vi "conversion_loop.vi"(0 "CAN frame array":T1[](array[typedef]) {"payload" format="%x"; "timestamp" format="%<%.7X\n%x>T"; "type" items=["CAN Data"=0, "CAN Remote"=1, "CAN Bus Error"=2, "CAN 2.0 Data"=8, "CAN FD Data"=16, "CAN FD+BRS Data"=24, "J1939 Data"=192, "Delay"=224, "Log Trigger"=225, "Start Trigger"=226]; "identifier" format="%x"}, 2 "CAN1 conversion session":T3, 3 "CAN2 conversion session":T3) -> (5 "CAN1 signal data":dbl[](array[numeric]), 6 "CAN2 signal data":dbl[](array[numeric]), 7 "CAN1 error out":errorcluster, 8 "CAN2 error out":errorcluster)   [LabVIEW 2017]
uses:
  <vilib>/xnet/xnet.llb/XNET Frame CAN.ctl
  <vilib>/xnet/xnet.llb/XNET Frame Type CAN.ctl
  <vilib>/xnet/xnet.llb/XNET Convert (Frame CAN to Signal).vi
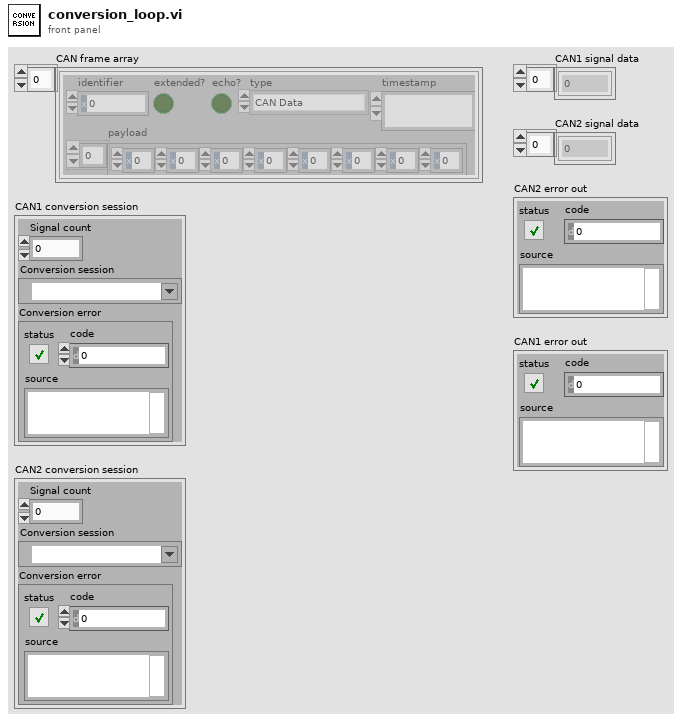
[diagram p1: front panel]
types:
  T1 = typedef "XNET Frame CAN.ctl" = cluster{"timestamp":timestamp, "payload":u8[], "identifier":u32, "type":T2, "extended?":bool, "echo?":bool}
  T2 = typedef "XNET Frame Type CAN.ctl" = u8
  T3 = cluster{"Signal count":i32, "Conversion session":refnum<k21>, "Conversion error":errorcluster}
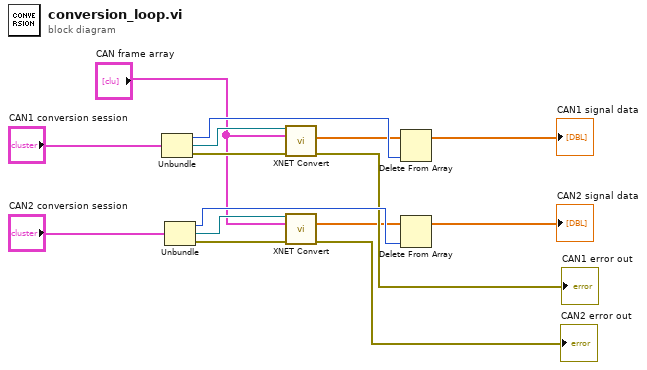
[diagram p0: block diagram]
diagram:
  n1 = Unbundle("CAN1 conversion session") -> ("Signal count"=w15:i32, "Conversion session"=w13:refnum<k21>, "Conversion error"=w10:errorcluster)
  n2 = Unbundle("CAN2 conversion session") -> ("Signal count"=w14:i32, "Conversion session"=w12:refnum<k21>, "Conversion error"=w11:errorcluster)
  n3 = call-poly <vilib>:"XNET Convert.vi"("session in"=w13, "frame data"="CAN frame array", "error in (no error)"=w10) -> ("signal data"=w1:dbl[], "error out"=→"CAN1 error out":errorcluster)  [unwired: 10 in, 1 out]
  n4 = call-poly <vilib>:"XNET Convert.vi"("session in"=w12, "frame data"="CAN frame array", "error in (no error)"=w11) -> ("signal data"=w2:dbl[], "error out"=→"CAN2 error out":errorcluster)  [unwired: 10 in, 1 out]
  n5 = Delete From Array(array=w1, index=w15) -> (array with subset deleted=→"CAN1 signal data":dbl[])  [unwired: 1 in, 1 out]
  n6 = Delete From Array(array=w2, index=w14) -> (array with subset deleted=→"CAN2 signal data":dbl[])  [unwired: 1 in, 1 out]
